vi "Get Identifier.vi"(8 "error in":errorcluster, 11 "NEOXID480HTA in":refnum<class "NEOXID480.lvclass">) -> (0 "error out":errorcluster, 2 "Identifier":string, 3 "NEOXID480HTA out":refnum<class "NEOXID480.lvclass">)   [LabVIEW 2024, in "NEOXID480.lvclass"]
uses:
  NEOXID480.lvclass
  NEOXID480.lvclass/NEOXID480.ctl
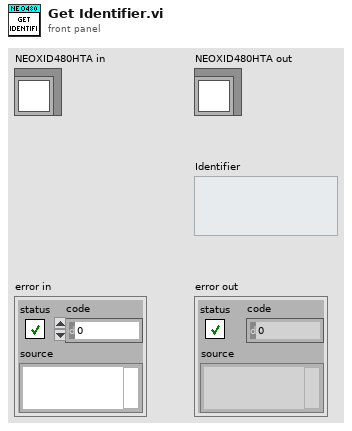
[diagram p1: front panel]
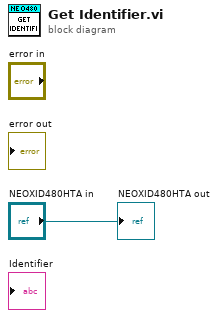
[diagram p0: block diagram]
diagram:
  "NEOXID480HTA out" <- "NEOXID480HTA in"
